vi "Force Sensor Main Loop.vi"(8 "error in (no error)":errorcluster, 9 "fs queue":refnum<queue>, 10 "fs notifier":refnum<notifier>, 11 "error queue":refnum<queue>) -> (0 "error out":errorcluster)   [LabVIEW 2020]
uses:
  GUI/Main GUI Loop/Handler.ctl
  Hardware/Sensors/Force Sensors/Force Sensor.lvclass
  C:/Users/jharw/Documents/1 Folder to Rule them All/UMD/Inflation-Apparatus/src/Hardware/General Hardware.lvclass
  Hardware/General Hardware.lvclass/General Hardware.ctl
  Hardware/General Hardware.lvclass
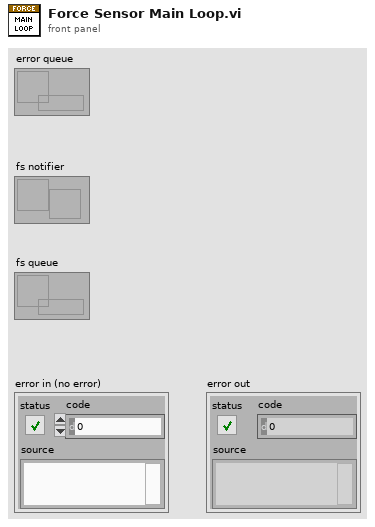
[diagram p1: front panel]
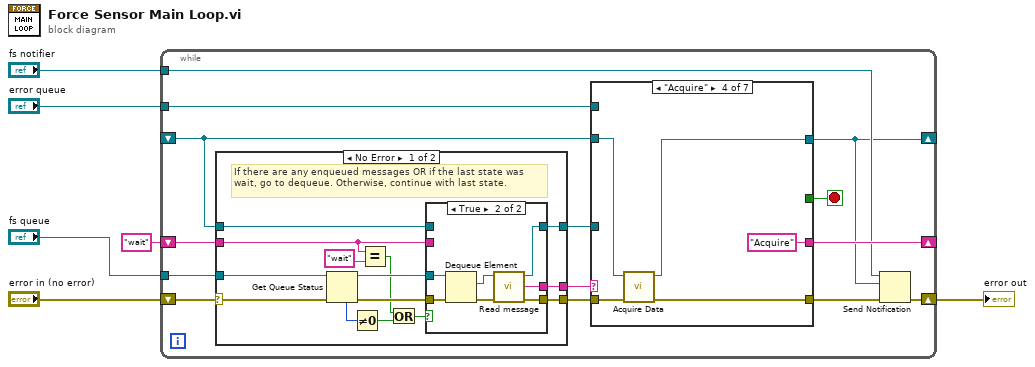
[diagram p0: block diagram]
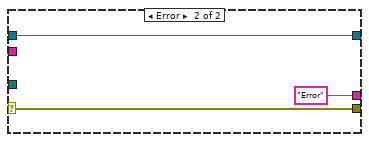
[diagram p3: hidden frame]
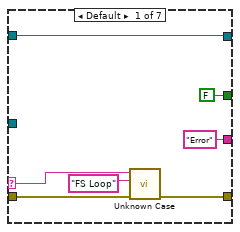
[diagram p4: hidden frame]
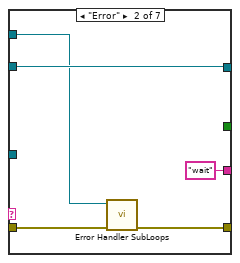
[diagram p5: hidden frame]
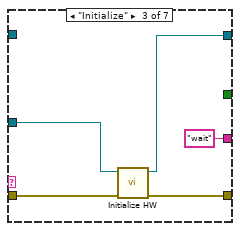
[diagram p6: hidden frame]
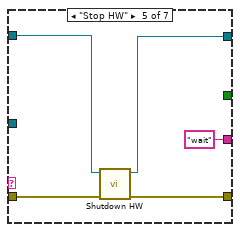
[diagram p7: hidden frame]
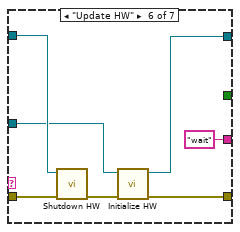
[diagram p8: hidden frame]
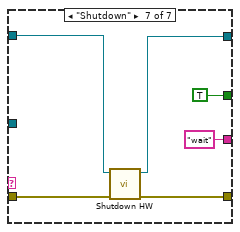
[diagram p9: hidden frame]
diagram:
  n1 = while {
    tunnel: "error queue" -> [w15]
    shift-right: [w9] -> w6
    shift-left: "error in (no error)" -> [w16]
    shift-right: [w17] -> _
    shift-left: "wait" -> [w20]
    shift-right: [w7] -> _
    shift-left: _ -> [w13]
    tunnel: "fs queue" -> [w11]
    tunnel: "fs notifier" -> [w8]
    stop <- w12 stop-if-true
    n2 = case shown="No Error" w16 {
      selector: w16 -> [w27 w47]
      tunnel: w20 -> [w31 _]
      tunnel: [w28 w47] -> w19
      tunnel: [w23 "Error" ("message")] -> w18
      tunnel: [w24 w45] -> w14
      tunnel: w13 -> [w22 w45]
      tunnel: w11 -> [w21 _]
      frame No Error {
        # "If there are any enqueued messages OR if the last state was wait, go to dequeue. Otherwise, continue with last state."
        n3 = Get Queue Status(queue=w21, error in (no error)=w27) -> (queue out=w34:refnum<queue>, error out=w33:errorcluster, # elements in queue=w26:i32)  [unwired: 1 in, 5 out]
        n4 = Not Equal To 0?(x=w26) -> (x != 0?=w25:bool)
        n5 = Equal?(x=w31, y="wait") -> (x = y?=w29:bool)
        n6 = Or(x=w29, y=w25) -> (x .or. y?=w32:bool)
        n7 = case shown="True" w32 {
          tunnel: w34 -> [_ w43]
          tunnel: w33 -> [w36 w44]
          tunnel: w31 -> [w37 _]
          tunnel: [w36 w40] -> w28
          tunnel: [w35 w39] -> w24
          tunnel: [w37 w38] -> w23
          tunnel: w22 -> [w35 _]
          frame False {
          }
          frame True {
            n8 = Dequeue Element(queue=w43, error in (no error)=w44) -> (element=w42:refnum<class "Force Sensor.lvclass">, error out=w41:errorcluster)  [unwired: 1 in, 2 out]
            n9 = call "Read message.vi"("error in (no error)"=w41, "General Hardware in"=w42) -> ("error out"=w40:errorcluster, "message"=w38:string, "General Hardware out"=w39:refnum<class "Force Sensor.lvclass">)  [unwired: 7 in]
          }
        }
      }
      frame Error {
      }
    }
    n10 = case shown="\"Acquire\"" w18 {
      selector: w18 -> [w52 _ _ _ _ _ _]
      tunnel: w19 -> [w54 w57 w63 w68 w73 w80 w85]
      tunnel: [w53 w56 w62 w65 w72 w78 w84] -> w10
      tunnel: ["Error" "wait" "wait" "Acquire" "wait" "wait" "wait"] -> w17
      tunnel: w15 -> [_ w55 _ _ _ _ _]
      tunnel: w14 -> [_ _ w60 _ _ w76 _]
      tunnel: [w49 w58 w61 w66 w70 w75 w82] -> w7
      tunnel: w13 -> [w49 w58 _ w67 w71 w77 w83]
      tunnel: [FALSE _ _ _ _ _ TRUE] -> w12
      frame Default {
        n11 = call "Unknown Case.vi"("error in (no error)"=w54, "source"="FS Loop", "case"=w52) -> ("error out"=w53:errorcluster)  [unwired: 8 in]
      }
      frame "Error" {
        n12 = call "Error Handler SubLoops.vi"("error in"=w57, "main gui queue"=w55) -> ("error out"=w56:errorcluster)  [unwired: 9 in]
      }
      frame "Initialize" {
        n13 = call-dynamic "Initialize HW.vi"("error in (no error)"=w63, "Force Sensor in"=w60) -> ("error out"=w62:errorcluster, "Force Sensor out"=w61:refnum<class "Force Sensor.lvclass">)  [unwired: 8 in]
      }
      frame "Acquire" {
        n14 = call-dynamic "Acquire Data.vi"("error in (no error)"=w68, "Force Sensor in"=w67) -> ("error out"=w65:errorcluster, "Force Sensor out"=w66:refnum<class "Force Sensor.lvclass">)  [unwired: 8 in]
      }
      frame "Stop HW" {
        n15 = call-dynamic "Shutdown HW.vi"("error in (no error)"=w73, "Force Sensor in"=w71) -> ("error out"=w72:errorcluster, "Force Sensor out"=w70:refnum<class "Force Sensor.lvclass">)  [unwired: 8 in]
      }
      frame "Update HW" {
        n16 = call-dynamic "Shutdown HW.vi"("error in (no error)"=w80, "Force Sensor in"=w77) -> ("error out"=w79:errorcluster)  [unwired: 8 in, 1 out]
        n17 = call-dynamic "Initialize HW.vi"("error in (no error)"=w79, "Force Sensor in"=w76) -> ("error out"=w78:errorcluster, "Force Sensor out"=w75:refnum<class "Force Sensor.lvclass">)  [unwired: 8 in]
      }
      frame "Shutdown" {
        n18 = call-dynamic "Shutdown HW.vi"("error in (no error)"=w85, "Force Sensor in"=w83) -> ("error out"=w84:errorcluster, "Force Sensor out"=w82:refnum<class "Force Sensor.lvclass">)  [unwired: 8 in]
      }
    }
    n19 = Send Notification(notification=w7, notifier=w8, error in (no error)=w10) -> (error out=w9:errorcluster)  [unwired: 1 out]
  }
  "error out" <- w6
